vi "Tester.vi"() -> ()   [LabVIEW 2017]
uses:
  <vilib>/ActorFramework/Message Enqueuer/Message Enqueuer.lvclass/Message Enqueuer.ctl
  Actors/Connection Listener/Connection Listener Messages/Get Connection List Msg/Get Connection List Msg.lvclass
  Applications/National Instruments/LabVIEW 2017 64-bit/vi.lib/ActorFramework/Reply Msg/Reply Msg.lvclass
  <vilib>/ActorFramework/Message Enqueuer/Message Enqueuer.lvclass
  <vilib>/ActorFramework/Reply Msg/Reply Msg.lvclass/Reply Msg.ctl
  Actors/Connection Listener/Connection Listener Messages/Forward Message Msg/Forward Message Msg.lvclass/Forward Message Msg.ctl
  <vilib>/ActorFramework/Message Enqueuer/Enqueue.vi
  Actors/Connection Listener/Connection Listener/Connection Listener.lvclass
  Applications/National Instruments/LabVIEW 2017 64-bit/vi.lib/ActorFramework/Actor/Actor.lvclass
  <vilib>/ActorFramework/Stop Msg/Stop Msg.lvclass
  Applications/National Instruments/LabVIEW 2017 64-bit/vi.lib/ActorFramework/Message/Message.lvclass
  <vilib>/ActorFramework/Reply Msg/Reply Msg.lvclass
  Actors/Connection Listener/Connection Listener Messages/Forward Message Msg/Forward Message Msg.lvclass
  <vilib>/ActorFramework/Message Priority Queue/Priority Enqueue.vi
  <vilib>/ActorFramework/Actor/Actor.lvclass
panel:
  in  "index":i32
  in  "client":bool
  in  "String":string
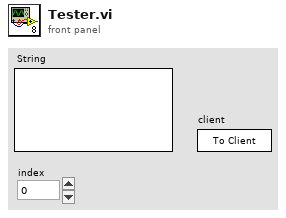
[diagram p1: front panel]
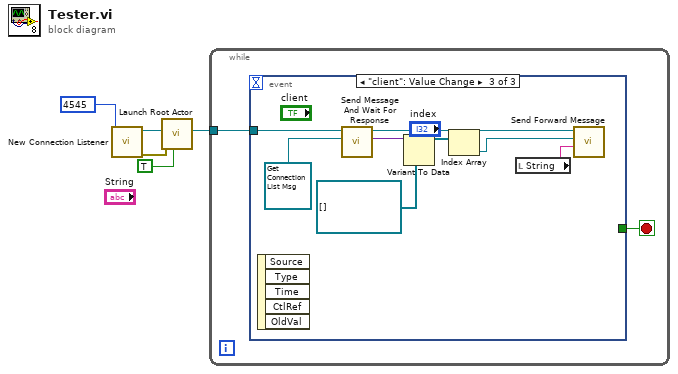
[diagram p0: block diagram]
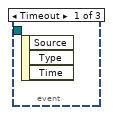
[diagram p2: hidden frame]
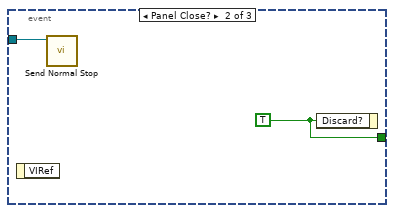
[diagram p3: hidden frame]
diagram:
  n1 = call "New Connection Listener.vi"("Port"=u16 4545) -> ("error out"=w3:errorcluster, "Connection Listener out"=w4:refnum<class "Connection Listener.lvclass">)  [unwired: 9 in]
  n2 = call <vilib>:"Launch Root Actor.vi"("Open Actor Core front panel? (F)"=TRUE, "error in (no error)"=w3, "Actor"=w4) -> ("Actor's Enqueuer"=w1:refnum<class "Message Enqueuer.lvclass">)  [unwired: 7 in, 1 out]
  n3 = while {
    tunnel: w1 -> [w6]
    stop <- w7 stop-if-true
    n4 = event shown="[2] \"client\": Value Change" {
      selector: _ -> [_ _ _]
      dyn-events: _ -> [_ _ _]
      timeout: _ -> [_ _ _]
      tunnel: [_ w9 _] -> w7
      tunnel: w6 -> [_ w8 w16]
      event Timeout {
        n5 = event-data() -> ()  [unwired: 1 in, 3 out]
      }
      event Panel Close? {
        w9 = TRUE ("Discard?")
        n6 = event-data() -> ()  [unwired: 1 in, 1 out]
        n7 = call <vilib>:"Send Normal Stop.vi"("Message Enqueuer"=w8) -> ()  [unwired: 10 in, 1 out]
        n8 = event-data("Discard?"=w9) -> ()  [unwired: 1 in, 1 out]
      }
      event "client": Value Change {
        n9 = event-data() -> ()  [unwired: 1 in, 5 out]
        n10 = call <vilib>:"Send Message And Wait For Response.vi"("Original Message"=refnum<class "Get Connection List Msg.lvclass"> refnum ("Connection Listener.lvlib:Get Connection List Msg.lvclass"), "Message Enqueuer in"=w16) -> ("Reply"=w14:variant)  [unwired: 6 in, 3 out]
        n11 = Variant To Data(type=refnum<class "Message Enqueuer.lvclass">[] [] ("ConnHandlers"), Variant=w14) -> (data=w12:refnum<class "Message Enqueuer.lvclass">[])  [unwired: 1 in, 1 out]
        n12 = Index Array(array=w12, index="index") -> (element=w11:refnum<class "Message Enqueuer.lvclass">)
        n13 = local read "String"() -> (w17:string)
        n14 = call "Send Forward Message.vi"("Message"=w17, "Dest Enqueuer"=w11, "Message Enqueuer in"=w16) -> ()  [unwired: 7 in, 2 out]
      }
    }
  }
